vi "Fetch Multi Eval Meas Trace IQ Constellation Results.vi"(8 "error in (no error)":errorcluster, 9 "Window Position (Low)":i32(ring) items=["Low", "High"], 10 "Instance (1)":T1=1, 11 "VISA resource name":refnum<visa-resource-name>) -> (0 "error out":errorcluster, 1 "I/Q Constellation Results":cluster{"I Phase":dbl, "Q Phase":dbl}[](array[cluster]) {"Q Phase" format="%^.3e"; "I Phase" format="%^.3e"}, 2 "Reliability":i32, 3 "VISA resource name out":refnum<visa-resource-name>)   [LabVIEW 2020, in "Rohde&Schwarz CMWXP NR FR1 Measurement.lvlib"]
doc: "Returns the results in the I/Q constellation diagram for low and high EVM window position. There is one pair of values per modulation symbol.\n\nAttributes:\nRSCMWXPNRFR1M_ATTR_FETCH_MULTI_EVAL_MEAS_TRACE_IQ_CONSTELLATION_LOW_RESULTS\nRSCMWXPNRFR1M_ATTR_FETCH_MULTI_EVAL_MEAS_TRACE_IQ_CONSTELLATION_HIGH_RESULTS\n\nRemote-control commands:\nFETCh:NRSub:MEAS<i>:MEValuation:TRACe:IQ:LOW?\nFETCh:NRSub:MEAS<i>:MEValuation:TRACe:IQ:HIGH?"
uses:
  <instrlib>/Rohde&Schwarz CMWXP NR FR1 Measurement/Rohde&Schwarz CMWXP NR FR1 Measurement.lvlib
  <instrlib>/Rohde&Schwarz CMWXP NR FR1 Measurement/Private/_Instance.ctl
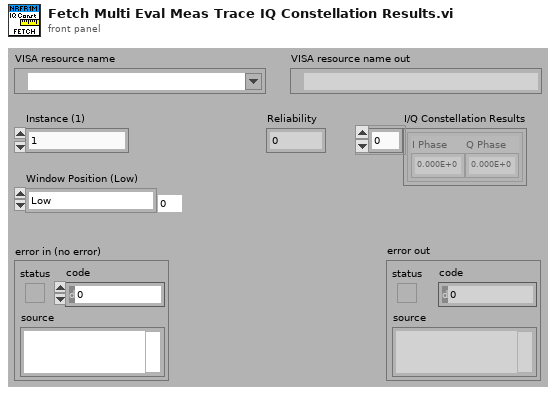
[diagram p1: front panel]
types:
  T1 = typedef "Rohde&Schwarz CMWXP NR FR1 Measurement.lvlib/_Instance.ctl" = i32
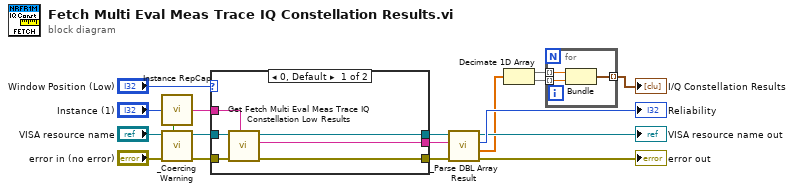
[diagram p0: block diagram]
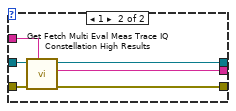
[diagram p2: hidden frame]
diagram:
  n1 = call <instrlib>:"Instance RepCap.vi"("Instance In"="Instance (1)") -> ("In Range?"=w15:bool, "RepCap Identifier Out"=w12:string)  [unwired: 1 in]
  n2 = call <instrlib>:"_Coercing Warning.vi"("In Range?"=w15, "error in (no error)"="error in (no error)", "VISA resource name"="VISA resource name") -> ("error out"=w13:errorcluster, "VISA resource name out"=w14:refnum<visa-resource-name>)  [unwired: 7 in]
  n3 = case shown="0, Default" "Window Position (Low)" {
    tunnel: w14 -> [w24 w30]
    tunnel: w13 -> [w23 w29]
    tunnel: w12 -> [w22 w28]
    tunnel: [w21 w27] -> w8
    tunnel: [w20 w26] -> w9
    tunnel: [w19 w25] -> w10
    frame 0, Default {
      n4 = call "Get Fetch Multi Eval Meas Trace IQ Constellation Low Results"("Repeated Capabilities"=w22, "error in (no error)"=w23, "instrument handle"=w24) -> ("error out"=w19:errorcluster, "Fetch Multi Eval Meas Trace IQ Constellation Low Results"=w20:string, "instrument handle out"=w21:refnum<visa-resource-name>)  [unwired: 6 in]
    }
    frame 1 {
      n5 = call "Get Fetch Multi Eval Meas Trace IQ Constellation High Results"("Repeated Capabilities"=w28, "error in (no error)"=w29, "instrument handle"=w30) -> ("error out"=w25:errorcluster, "Fetch Multi Eval Meas Trace IQ Constellation High Results"=w26:string, "instrument handle out"=w27:refnum<visa-resource-name>)  [unwired: 6 in]
    }
  }
  n6 = call <instrlib>:"_Parse DBL Array Result.vi"("error in (no error)"=w10, "Input String"=w9, "VISA resource name"=w8) -> ("error out"=→"error out":errorcluster, "Results"=w4:dbl[], "Reliability"=→"Reliability":i32, "VISA resource name out"=→"VISA resource name out":refnum<visa-resource-name>)  [unwired: 5 in]
  n7 = Decimate 1D Array(w4) -> (w3:dbl[], w2:dbl[])
  n8 = for {
    tunnel: w3 -> [w33] mode=indexing
    tunnel: w2 -> [w32] mode=indexing
    tunnel: [w31] -> w1 mode=indexing
    n9 = Bundle("Element"=w33, "Element"=w32) -> (w31:cluster{"Element":dbl, "Element":dbl})  [unwired: 1 in]
  }
  "I/Q Constellation Results" <- w1
